vi "Get Discovery Service Key File Path.vi"(8 "error in":errorcluster, 11 "cluster id (\"\")":string) -> (0 "error out":errorcluster, 3 "key file path":path)   [LabVIEW 2020, in "Plug-In SDK Discovery V1 API.lvlib"]
uses:
  Plug-In SDK Discovery V1 API.lvlib
  <vilib>/Utility/sysdir.llb/System Directory Type.ctl
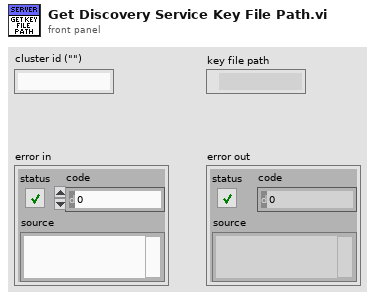
[diagram p1: front panel]
types:
  T1 = typedef "System Directory Type.ctl" = i32
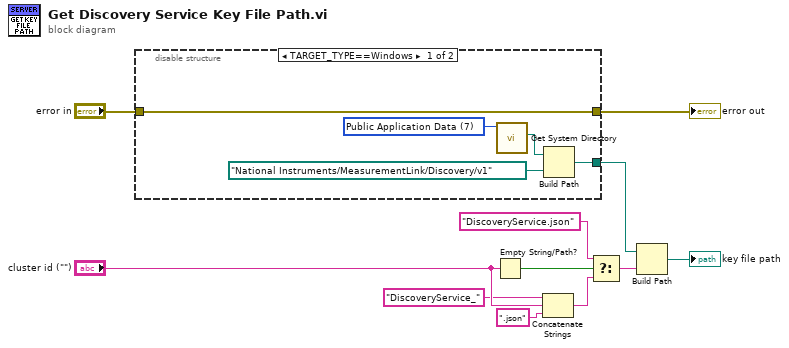
[diagram p0: block diagram]
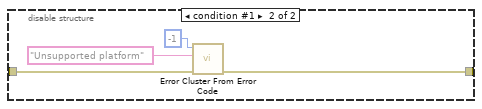
[diagram p2: hidden frame]
diagram:
  n1 = disable-structure shown="TARGET_TYPE==Windows" {
    disable-tunnel: [w13 _] -> w6
    disable-tunnel: "error in" -> [w12 w18]
    disable-tunnel: [w12 w17] -> w11
    frame condition #0 (active) {
      w16 = T1 7 items=["User Home"=0, "User Desktop"=1, "User Documents"=2, "User Application Data"=3, "User Preferences"=4, "User Temporary"=5, "Public Documents"=6, "Public Application Data"=7, "Public Preferences"=8, "Public Cache"=13, "System Core Libraries"=9, "System Installed Libraries"=10, "Application Files"=11, "Boot Volume Root"=12] ("system directory type")
      n2 = call <vilib>:"Get System Directory.vi"("system directory type"=w16) -> ("system directory"=w15:path)  [unwired: 10 in]
      n3 = Build Path(base path=w15, name or relative path=path "National Instruments/MeasurementLink/Discovery/v1") -> (appended path=w13:path)
    }
    frame condition #1 {
      n4 = call <vilib>:"Error Cluster From Error Code.vi"("error in (no error)"=w18, "error message (\"\")"="Unsupported platform" ("error message (\"\")"), "error code (0)"=-1) -> ("error out"=w17:errorcluster)  [unwired: 6 in]
    }
  }
  "error out" <- w11
  n5 = Empty String/Path?(string/path="cluster id (\"\")") -> (empty?=w4:bool)
  n6 = Concatenate Strings("DiscoveryService_", "cluster id (\"\")", ".json") -> (w5:string)
  n7 = Select(t="DiscoveryService.json", s=w4, f=w5) -> (s? t:f=w7:string)
  n8 = Build Path(base path=w6, name or relative path=w7) -> (appended path=→"key file path":path)
